vi "HCC Cycle Count Filter.vi"(8 "Error In":errorcluster, 10 "Incoming Cycle Count":u16, 11 "Diagnostic":T1) -> (0 "Error Out":errorcluster, 3 "Filtered Cycle Count":u16, 5 "Elapsed Time (sec)":dbl format="%.2f")   [LabVIEW 2016]
uses:
  Type Definitions/ViperHawk/ViperHawk Diagnostic Data.ctl
  <vilib>/ptbypt/NI_PtbyPt.lvlib
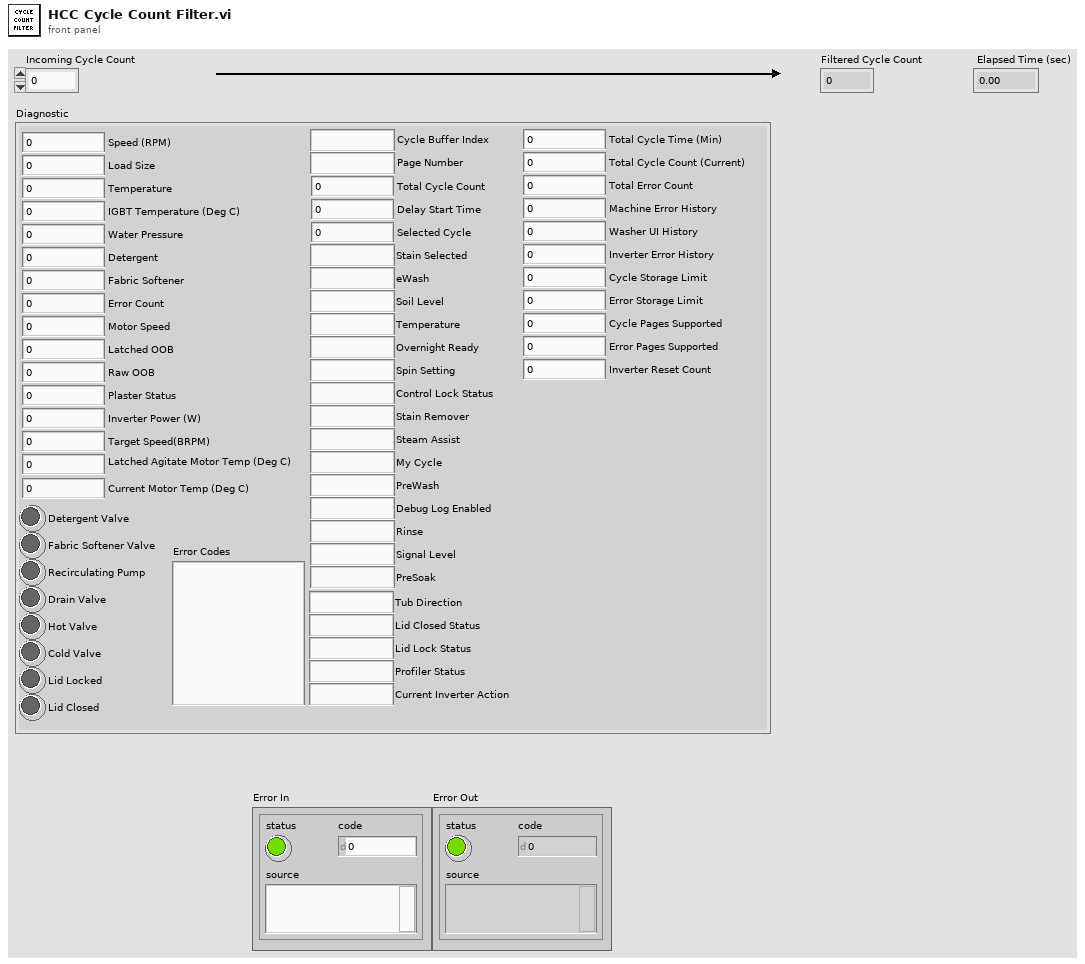
[diagram p1: front panel]
types:
  T1 = typedef "ViperHawk Diagnostic Data.ctl" = cluster{"Speed (RPM)":u32, "Load Size":u32, "Temperature":u32, "Water Pressure":dbl, "Detergent":u32, "Fabric Softener":u32, "Tub Direction":string, "Detergent Valve":bool, "Fabric Softener Valve":bool, "Recirculating Pump":bool, "Drain Valve":bool, "Hot Valve":bool, "Cold Valve":bool, "Lid Closed Status":string, "Lid Lock Status":string, "Error Count":u32, "IGBT Temperature (Deg C)":u32, "Motor Speed":u32, "Latched OOB":u32, "Raw OOB":u32, "Plaster Status":u32, "Inverter Power (W)":u32, "Target Speed(BRPM)":u32, "Latched Agitate Motor Temp (Deg C)":u32, "Current Motor Temp (Deg C)":u32, "Profiler Status":string, "Current Inverter Action":string, "Error Codes":string, "Lid Locked":bool, "Lid Closed":bool, "9E Diagnostic Data":cluster{"Total Cycle Time (Min)":u32, "Total Cycle Count (Current)":u16, "Total Error Count":u16, "Machine Error History":u32, "Washer UI History":u32, "Inverter Error History":u32, "Cycle Storage Limit":u8, "Error Storage Limit":u8, "Cycle Pages Supported":u8, "Error Pages Supported":u8, "Inverter Reset Count":u16}, "9F Diagnostic Data":cluster{"Cycle Buffer Index":string, "Page Number":string, "Total Cycle Count":u32, "Delay Start Time":u32, "Stain Selected":string, "Selected Cycle":u32, "eWash":string, "Soil Level":string, "Temperature":string, "Overnight Ready":string, "Spin Setting":string, "Control Lock Status":string, "Stain Remover":string, "Steam Assist":string, "My Cycle":string, "PreWash":string, "Debug Log Enabled":string, "Rinse":string, "Signal Level":string, "PreSoak":string}}
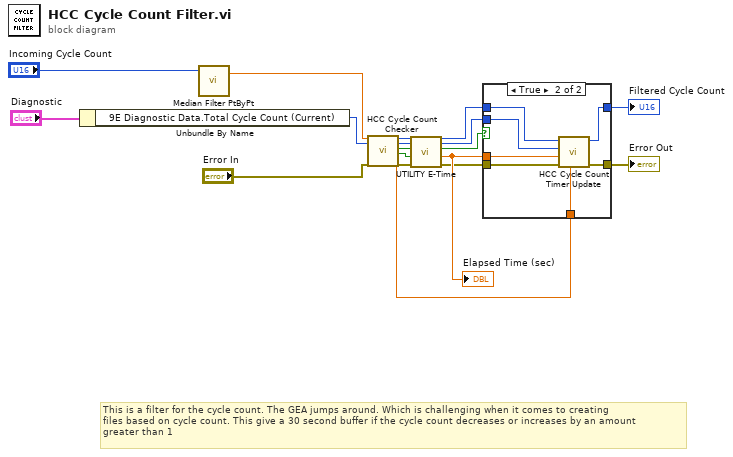
[diagram p0: block diagram]
diagram:
  # "This is a filter for the cycle count. The GEA jumps around. Which is challenging when it comes to creating\nfiles based on cycle count. This give a 30 second buffer if the cycle count decreases or increases by an amount \ngreater than 1"
  n1 = Unbundle By Name("Diagnostic") -> ("9E Diagnostic Data.Total Cycle Count (Current)"=w10:u16)
  n2 = call <vilib>:"Median Filter PtByPt.vi"("x"="Incoming Cycle Count") -> ("Filtered x"=w11:dbl)  [unwired: 3 in, 1 out]
  n3 = call "HCC Cycle Count Checker.vi"("Input Cycle Count"=w11, "Total Cycle Count (Current)"=w10, "Error In"="Error In") -> ("Input Cycle Count OUT"=w7:u16, "Total Cycle Count (Current) OUT"=w6:u16, "Enter Timer Loop"=w9:bool, "Reset Timer"=w8:bool, "Timer Limit"=w3:dbl, "Error Out"=w1:errorcluster)  [unwired: 11 in]
  n4 = call "UTILITY E-Time.vi"("error in (no error)"=w1, "Reset"=w8) -> ("error out"=w5:errorcluster, "Elapsed Time (sec)"=w12:dbl)  [unwired: 7 in, 1 out]
  "Elapsed Time (sec)" <- w12
  n5 = case shown="True" w9 {
    tunnel: w6 -> [_ w24]
    tunnel: [w17 w23] -> w13
    tunnel: w7 -> [w17 w21]
    tunnel: w12 -> [_ w22]
    tunnel: w5 -> [w16 w20]
    tunnel: [w16 w19] -> w4
    tunnel: w3 -> [_ w18]
    frame False {
    }
    frame True {
      n6 = call "HCC Cycle Count Timer Update.vi"("Timer Limit"=w18, "Error In"=w20, "Elapsed Time (sec)"=w22, "Total Cycle Count (Current) OUT"=w24, "Input Cycle Count OUT in"=w21) -> ("Error Out"=w19:errorcluster, "Input Cycle Count OUT out"=w23:u16)  [unwired: 5 in]
    }
  }
  "Filtered Cycle Count" <- w13
  "Error Out" <- w4
